vi "ORS_InvertFunction.vi"(2 "Rescale to input":bool, 3 "input":dbl[](array[numeric]) caption="Hilbert in", 4 "number of points":i32, 5 "method":i32(ring)=2 items=["nearest", "linear", "spline", "cubic Hermite", "Lagrange"]) -> (1 "inverted output":dbl[](array[numeric]))   [LabVIEW 2024]
uses:
  <vilib>/Analysis/1siggen.llb/Ramp Pattern by Samples.vi
  <vilib>/gmath/NI_Gmath.lvlib
  <vilib>/Analysis/NI_AALBase.lvlib
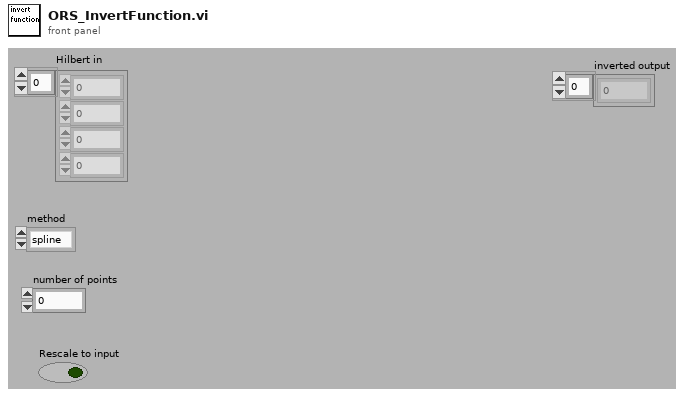
[diagram p1: front panel]
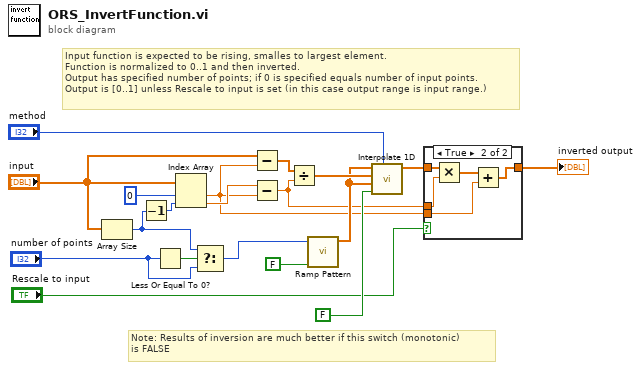
[diagram p0: block diagram]
diagram:
  # "Note: Results of inversion are much better if this switch (monotonic) \nis FALSE"
  # "Input function is expected to be rising, smalles to largest element.\nFunction is normalized to 0..1 and then inverted.\nOutput has specified number of points; if 0 is specified equals number of input points.\nOutput is [0..1] unless Rescale to input is set (in this case output range is input range.)"
  n1 = Array Size(array="input") -> (size(s)=w7:i32)
  n2 = Decrement(x=w7) -> (x-1=w18:i32)
  n3 = Less Or Equal To 0?(x="number of points") -> (x <= 0?=w8:bool)
  n4 = Index Array(array="input", index #1=0 ("index"), index #2=w18) -> (element #1=w3:dbl, element #2=w16:dbl)
  n5 = Select(t=w7, s=w8, f="number of points") -> (s? t:f=w9:i32)
  n6 = Subtract(x="input", y=w3) -> (x-y=w15:dbl[])
  n7 = Subtract(x=w16, y=w3) -> (x-y=w4:dbl)
  n8 = Divide(x=w15, y=w4) -> (x/y=w14:dbl[])
  n9 = call-poly <vilib>:"Ramp Pattern.vi"("exclude end?"=FALSE, "samples"=w9) -> ("Ramp Pattern"=w13:dbl[])  [unwired: 8 in, 1 out]
  n10 = call <vilib>:"Interpolate 1D.vi"("method"="method", "X is monotonic"=FALSE, "xi"=w13, "X"=w14, "Y"=w13) -> ("yi"=w5:dbl[])  [unwired: 4 in, 2 out]
  n11 = case shown="True" "Rescale to input" {
    tunnel: w5 -> [w20 w25]
    tunnel: w4 -> [_ w24]
    tunnel: w3 -> [_ w22]
    tunnel: [w20 w21] -> w2
    frame False {
    }
    frame True {
      n12 = Multiply(x=w25, y=w24) -> (x*y=w23:dbl[])
      n13 = Add(x=w23, y=w22) -> (x+y=w21:dbl[])
    }
  }
  "inverted output" <- w2
